vi "UTIL Update Median Filter.vi"(8 "Error In":errorcluster, 10 "Data Point":dbl, 11 "Average Queue":refnum<queue>) -> (0 "Error Out":errorcluster, 3 "Moving Average (dB)":dbl)   [LabVIEW 2010]
doc: "This computes a backward Moving Average, using a fixed-length Queue to hold the last N points. The algorithm is simple -- do a Lossy Enqueue, which bumps out the oldest point, use the Get Queue Status to get the Queue contents (without emptying the Queue) and return the Mean.\n\nInput:\n Average Qyeye Fixed-length Queue of Dbl\n DataPoint Dbl\n Error In\nOutput:\n Moving Average Dbl\n Error Out"
uses:
  <vilib>/Analysis/NI_AALBase.lvlib
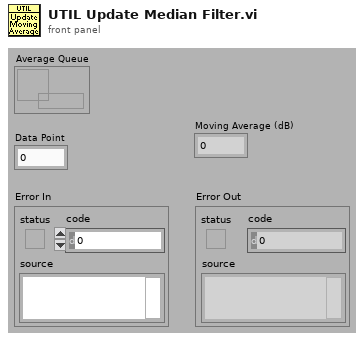
[diagram p1: front panel]
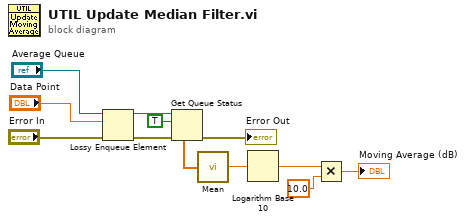
[diagram p0: block diagram]
diagram:
  n1 = Lossy Enqueue Element(queue="Average Queue", element="Data Point", error in (no error)="Error In") -> (queue out=w7:refnum<queue>, error out=w11:errorcluster)  [unwired: 2 out]
  n2 = Get Queue Status(queue=w7, return elements? (F)=TRUE, error in (no error)=w11) -> (error out=→"Error Out":errorcluster, elements=w5:dbl[])  [unwired: 6 out]
  n3 = call <vilib>:"Mean.vi"("X"=w5) -> ("mean"=w4:dbl)  [unwired: 1 out]
  n4 = Logarithm Base 10(1:w4) -> (0:w3:dbl)
  n5 = Multiply(x=w3, y=10.0) -> (x*y=→"Moving Average (dB)":dbl)
